vi "List of Folder Number of Elements - Indices.vi"(11 "# Elements Array":i32[](array[numeric])) -> (3 "Output String":string)   [LabVIEW 2021, in "Strings.lvlib"]
uses:
  Strings.lvlib
  <userlib>/_OpenG.lib/array/array.llb/Remove Duplicates from 1D Array (I32)__ogtk.vi
  <userlib>/_OpenG.lib/array/array.llb/Filter 1D Array with Scalar (I32)__ogtk.vi
  <userlib>/_OpenG.lib/array/array.llb/openg_array.lvlib
panel:
  # "if there are more than one # Elements, outputs a table of:\n# Elements, list of indices"
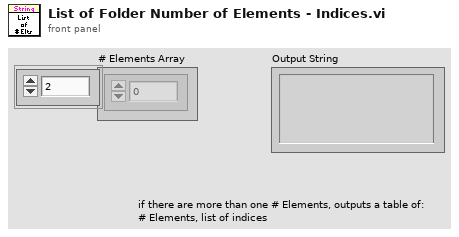
[diagram p1: front panel]
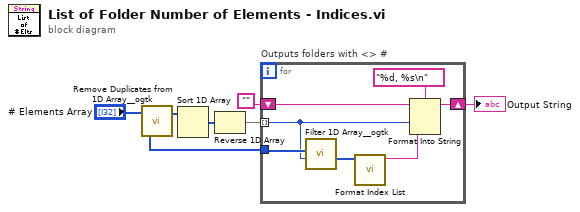
[diagram p0: block diagram]
diagram:
  n1 = call-poly <userlib>:"Remove Duplicates from 1D Array__ogtk.vi"("Input Array"="# Elements Array") -> ("Output Array"=w3:i32[])  [unwired: 1 out]
  n2 = Sort 1D Array(array=w3) -> (sorted array=w4:i32[])
  n3 = Reverse 1D Array(array=w4) -> (reversed array=w5:i32[])
  n4 = for "Outputs folders with <> #" {
    tunnel: "# Elements Array" -> [w13]
    tunnel: w5 -> [w10] mode=indexing
    shift-right: [w7] -> w1
    shift-left: "" -> [w8]
    n5 = call-poly <userlib>:"Filter 1D Array__ogtk.vi"("items to filter"=w10, "array"=w13) -> ("filtered item indices"=w12:i32[])  [unwired: 4 in, 1 out]
    n6 = call "Format Index List.vi"("Index Array"=w12) -> ("Index List"=w11:string)  [unwired: 10 in]
    n7 = Format Into String(format string="%d, %s\n", initial string=w8, w10, w11) -> (resulting string=w7:string)  [unwired: 1 in, 1 out]
  }
  "Output String" <- w1
